vi "Write Logger.vi"(8 "error in (no error)":errorcluster, 10 "Logger":T1, 11 "Log Message in":refnum<class "Log Message.lvclass">) -> (0 "error out":errorcluster, 3 "Log Message out":refnum<class "Log Message.lvclass">)   [LabVIEW 2024, in "AIM ARINC 429 Engine.lvlib" / "Implementation.lvlib" / "Word Logging.lvlib" / "Log Message.lvclass"]
uses:
  Log Message.lvclass
  Logger Data Reference.ctl
  Logger Interface/Logger Interface.lvclass
  Log Message.lvclass/Log Message.ctl
  Word Logging.lvlib
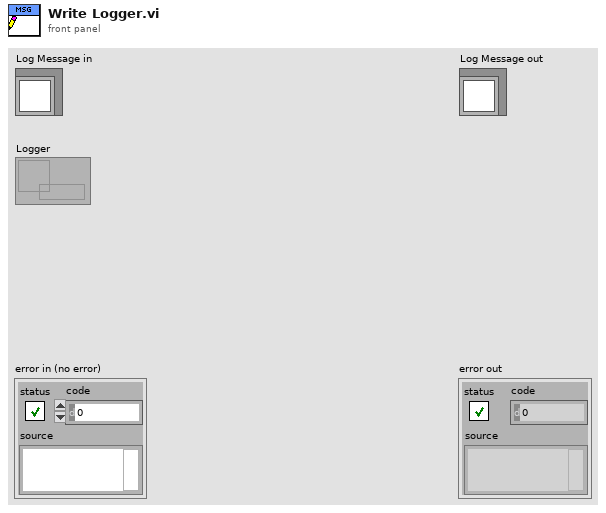
[diagram p1: front panel]
types:
  T1 = typedef "AIM ARINC 429 Engine.lvlib/Implementation.lvlib/Word Logging.lvlib/Logger Data Reference.ctl" = refnum<data-value>
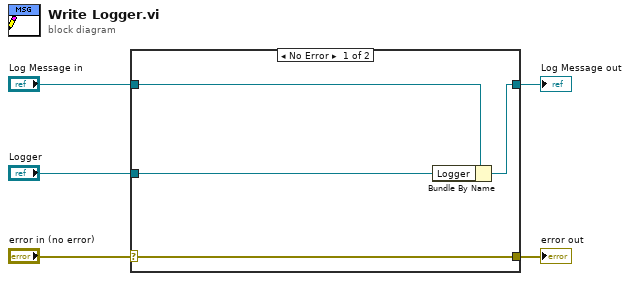
[diagram p0: block diagram]
diagram:
  n1 = case shown="No Error" "error in (no error)" {
    selector: "error in (no error)" -> [w9 w10]
    tunnel: [w9 w10] -> w4
    tunnel: [w7 w11] -> w2
    tunnel: "Log Message in" -> [w8 w11]
    tunnel: "Logger" -> [w6 _]
    frame No Error {
      n2 = Bundle By Name(cluster=w8, "Logger"=w6) -> (w7:refnum<class "Log Message.lvclass">)
    }
    frame Error {
    }
  }
  "error out" <- w4
  "Log Message out" <- w2
